vi "Init2.vi"(0 "ClassWriterNative.lvclass":refnum<class "ClassWriterNative.lvclass">, 1 "LvClassRef":refnum<vi>, 5 "error in (no error)":errorcluster) -> (14 "ClassWriterNative.lvclass":refnum<class "ClassWriterNative.lvclass">, 19 "error out":errorcluster)   [LabVIEW 2020, in "ClassWriterNative.lvclass"]
uses:
  ClassWriterNative.lvclass
  C:/Program Files (x86)/National Instruments/LabVIEW 2020/resource/Framework/Providers/Open_GDS/ClassProviders/Provider_BaseClassInterface/ClassWriter_class/ClassWriter.lvclass
  ClassWriterNative.lvclass/ClassWriterNative.ctl
  Provider_BaseClassInterface/ClassWriter_class/ClassWriter.lvclass
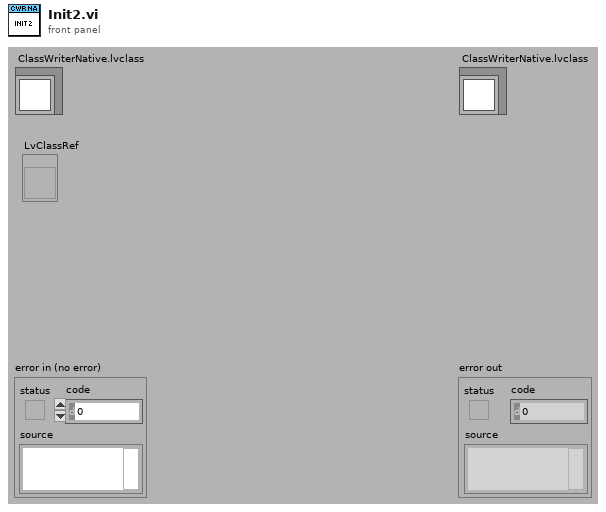
[diagram p1: front panel]
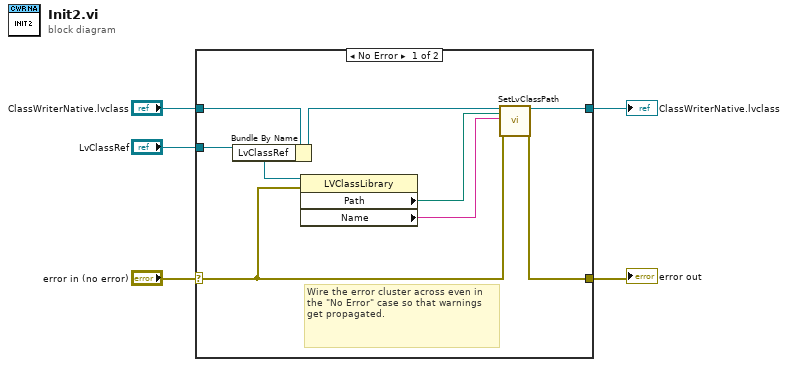
[diagram p0: block diagram]
diagram:
  n1 = case shown="No Error" "error in (no error)" {
    selector: "error in (no error)" -> [w7 w15]
    tunnel: [w6 w15] -> w4
    tunnel: [w11 w14] -> w2
    tunnel: "ClassWriterNative.lvclass" -> [w13 w14]
    tunnel: "LvClassRef" -> [w10 _]
    frame No Error {
      # "Wire the error cluster across even in the \"No Error\" case so that warnings get propagated."
      n2 = Bundle By Name(cluster=w13, "LvClassRef"=w10) -> (w12:refnum<class "ClassWriterNative.lvclass">)
      n3 = property class="LVClassLibrary"(reference=w10, error in=w7) -> ("Path"=w9:path, "Name"=w8:string)  [unwired: 2 out]
      n4 = call "SetLvClassPath.vi"("ClassWriter"=w12, "ClassPath"=w9, "ClassName"=w8, "error in (no error)"=w7) -> ("ClassWriter"=w11:refnum<class "ClassWriterNative.lvclass">, "error out"=w6:errorcluster)  [unwired: 14 in]
    }
    frame Error {
    }
  }
  "error out" <- w4
  "ClassWriterNative.lvclass" <- w2
